vi "Configuracao.Escrita.vi"(8 "error in (no error)":errorcluster) -> (0 "error out":errorcluster)   [LabVIEW 2019]
uses:
  Configuracao.Variaveis.vi
  TelaParametrosTeste/VariaveisParametros.vi
  Relatorio/Relatorio_Variaveis.vi
  <vilib>/Utility/xml.llb/Write to XML File(string).vi
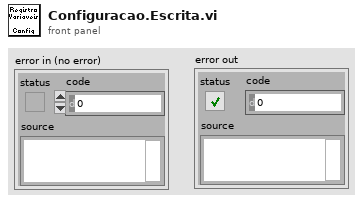
[diagram p1: front panel]
types:
  T1 = enum16{"None", "Continua", "Senoidal", "Quadrada"}
  T2 = cluster{"PicoRotacaoMax":dbl, "PicoRotacaoMin":dbl, "RotacoesMinuto":dbl}
  T3 = cluster{"TempRampas":dbl, "PicoMax":dbl, "TextUnidMed":string}
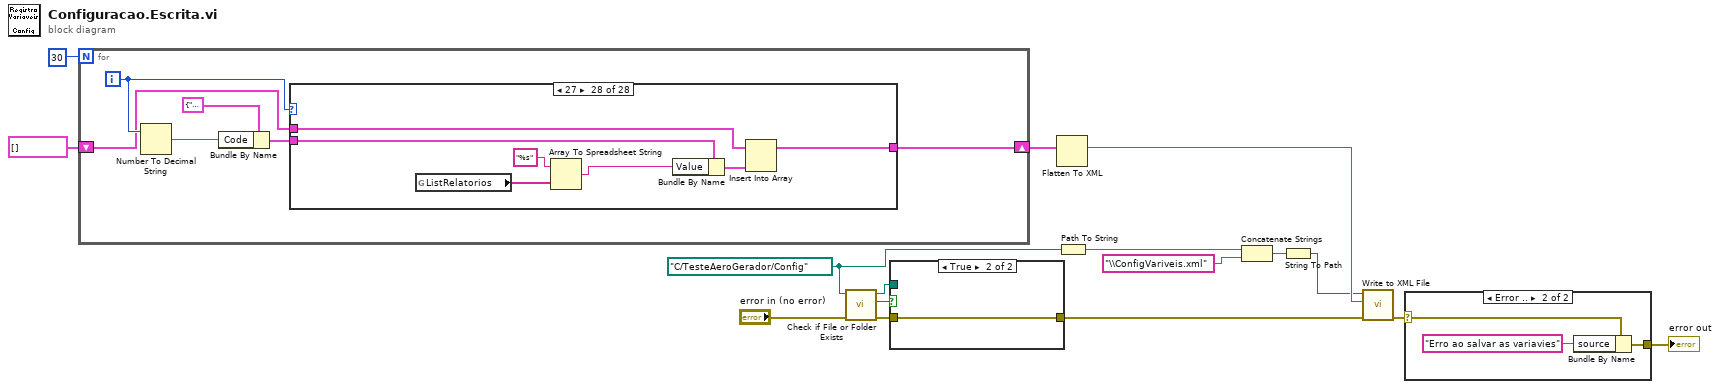
[diagram p0: block diagram]
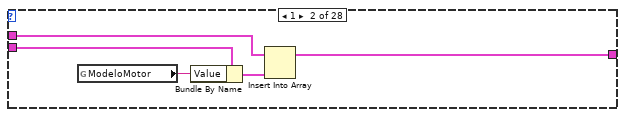
[diagram p4: hidden frame]
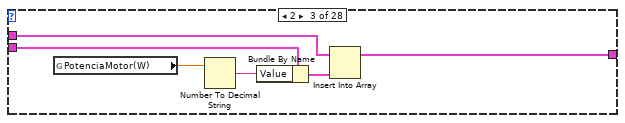
[diagram p5: hidden frame]
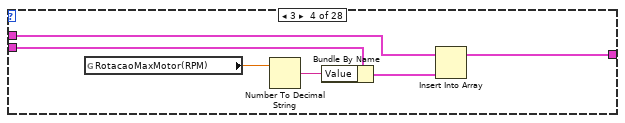
[diagram p6: hidden frame]
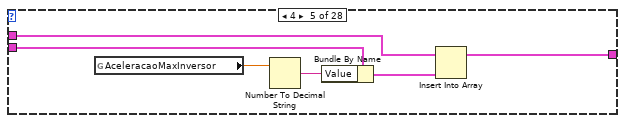
[diagram p7: hidden frame]
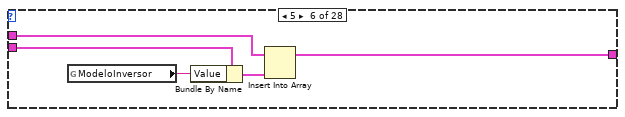
[diagram p8: hidden frame]
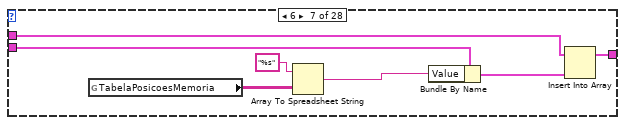
[diagram p9: hidden frame]
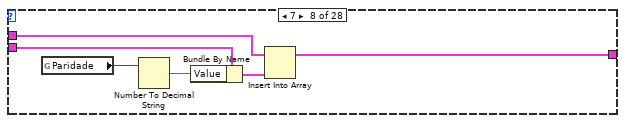
[diagram p10: hidden frame]
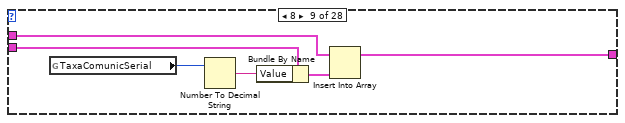
[diagram p11: hidden frame]
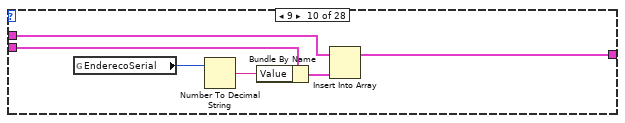
[diagram p12: hidden frame]
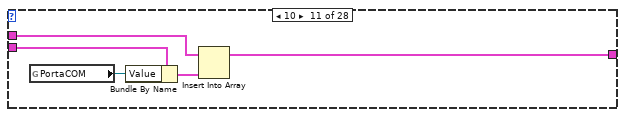
[diagram p13: hidden frame]
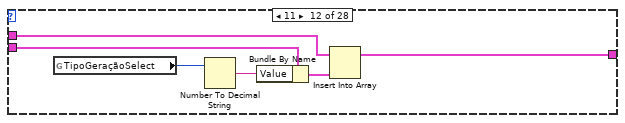
[diagram p14: hidden frame]
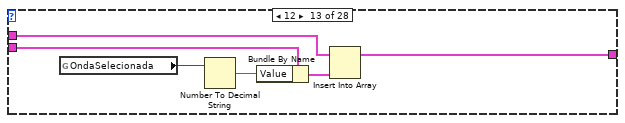
[diagram p15: hidden frame]
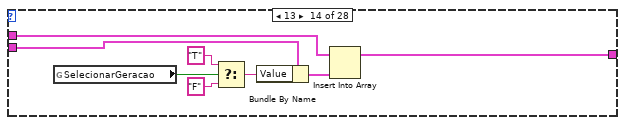
[diagram p16: hidden frame]
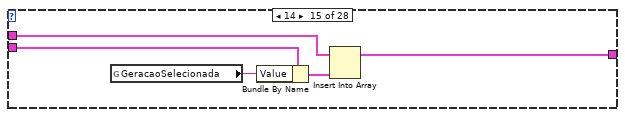
[diagram p17: hidden frame]
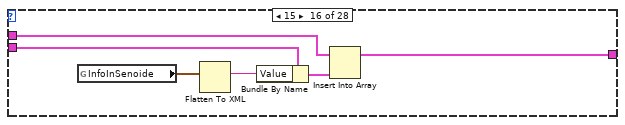
[diagram p18: hidden frame]
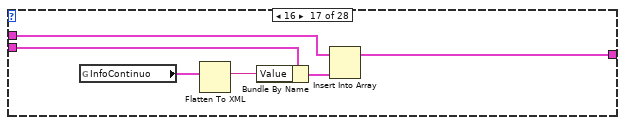
[diagram p19: hidden frame]
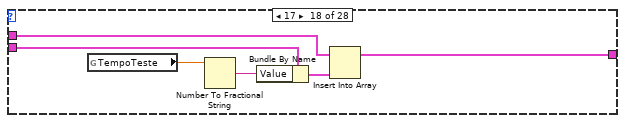
[diagram p20: hidden frame]
diagram:
  w11 = path "C:/TesteAeroGerador/Config" ("XML File Path")
  n1 = for {
    N: 30 -> [_]
    shift-right: [w18] -> w3
    shift-left: cluster{"Code":string, "Value":string}[] [] -> [w19]
    i -> [w20]
    n2 = Number To Decimal String(number=w20) -> (decimal integer string=w21:string)  [unwired: 1 in]
    n3 = Bundle By Name(cluster=cluster{"Code":string, "Value":string} {"Code"="", "Value"=""} ("output cluster"), "Code"=w21) -> (w17:cluster{"Code":string, "Value":string})
    n4 = case shown="27" w20 {
      tunnel: w19 -> [w23 w28 w34 w40 w46 w51 w58 w64 w70 w76 w81 w87 w93 w101 w106 w112 w118 w124 w131 w139 w145 w151 w157 w163 w169 w174 w176 w185]
      tunnel: [w23 w27 w33 w39 w45 w50 w57 w63 w69 w75 w80 w86 w92 w100 w105 w111 w117 w123 w130 w138 w144 w150 w156 w162 w168 w173 w175 w184] -> w18
      tunnel: w17 -> [_ w26 w32 w38 w44 w49 w56 w62 w68 w74 w79 w85 w91 w99 w104 w110 w116 w122 w129 w137 w143 w149 w155 w161 w167 w172 w177 w186]
      frame 0, Default {
      }
      frame 1 {
        n5 = global read "Configuracao.Variaveis.vi" "ModeloMotor"() -> (w25:string)
        n6 = Bundle By Name(cluster=w26, "Value"=w25) -> (w24:cluster{"Code":string, "Value":string})
        n7 = Insert Into Array(array=w28, new element=w24) -> (w27:cluster{"Code":string, "Value":string}[])  [unwired: 1 in]
      }
      frame 2 {
        n8 = global read "Configuracao.Variaveis.vi" "PotenciaMotor(W)"() -> (w30:dbl)
        n9 = Number To Decimal String(number=w30) -> (decimal integer string=w29:string)  [unwired: 1 in]
        n10 = Bundle By Name(cluster=w32, "Value"=w29) -> (w31:cluster{"Code":string, "Value":string})
        n11 = Insert Into Array(array=w34, new element=w31) -> (w33:cluster{"Code":string, "Value":string}[])  [unwired: 1 in]
      }
      frame 3 {
        n12 = global read "Configuracao.Variaveis.vi" "RotacaoMaxMotor(RPM)"() -> (w36:dbl)
        n13 = Number To Decimal String(number=w36) -> (decimal integer string=w35:string)  [unwired: 1 in]
        n14 = Bundle By Name(cluster=w38, "Value"=w35) -> (w37:cluster{"Code":string, "Value":string})
        n15 = Insert Into Array(array=w40, new element=w37) -> (w39:cluster{"Code":string, "Value":string}[])  [unwired: 1 in]
      }
      frame 4 {
        n16 = global read "Configuracao.Variaveis.vi" "AceleracaoMaxInversor"() -> (w42:dbl)
        n17 = Number To Decimal String(number=w42) -> (decimal integer string=w41:string)  [unwired: 1 in]
        n18 = Bundle By Name(cluster=w44, "Value"=w41) -> (w43:cluster{"Code":string, "Value":string})
        n19 = Insert Into Array(array=w46, new element=w43) -> (w45:cluster{"Code":string, "Value":string}[])  [unwired: 1 in]
      }
      frame 5 {
        n20 = global read "Configuracao.Variaveis.vi" "ModeloInversor"() -> (w47:string)
        n21 = Bundle By Name(cluster=w49, "Value"=w47) -> (w48:cluster{"Code":string, "Value":string})
        n22 = Insert Into Array(array=w51, new element=w48) -> (w50:cluster{"Code":string, "Value":string}[])  [unwired: 1 in]
      }
      frame 6 {
        n23 = global read "Configuracao.Variaveis.vi" "TabelaPosicoesMemoria"() -> (w53:string[][])
        n24 = Array To Spreadsheet String(array=w53, 3:"%s" ("format string")) -> (spreadsheet string=w52:string)  [unwired: 1 in]
        n25 = Bundle By Name(cluster=w56, "Value"=w52) -> (w55:cluster{"Code":string, "Value":string})
        n26 = Insert Into Array(array=w58, new element=w55) -> (w57:cluster{"Code":string, "Value":string}[])  [unwired: 1 in]
      }
      frame 7 {
        n27 = global read "Configuracao.Variaveis.vi" "Paridade"() -> (w60:u16)
        n28 = Number To Decimal String(number=w60) -> (decimal integer string=w59:string)  [unwired: 1 in]
        n29 = Bundle By Name(cluster=w62, "Value"=w59) -> (w61:cluster{"Code":string, "Value":string})
        n30 = Insert Into Array(array=w64, new element=w61) -> (w63:cluster{"Code":string, "Value":string}[])  [unwired: 1 in]
      }
      frame 8 {
        n31 = global read "Configuracao.Variaveis.vi" "TaxaComunicSerial"() -> (w66:u32)
        n32 = Number To Decimal String(number=w66) -> (decimal integer string=w65:string)  [unwired: 1 in]
        n33 = Bundle By Name(cluster=w68, "Value"=w65) -> (w67:cluster{"Code":string, "Value":string})
        n34 = Insert Into Array(array=w70, new element=w67) -> (w69:cluster{"Code":string, "Value":string}[])  [unwired: 1 in]
      }
      frame 9 {
        n35 = global read "Configuracao.Variaveis.vi" "EnderecoSerial"() -> (w72:u8)
        n36 = Number To Decimal String(number=w72) -> (decimal integer string=w71:string)  [unwired: 1 in]
        n37 = Bundle By Name(cluster=w74, "Value"=w71) -> (w73:cluster{"Code":string, "Value":string})
        n38 = Insert Into Array(array=w76, new element=w73) -> (w75:cluster{"Code":string, "Value":string}[])  [unwired: 1 in]
      }
      frame 10 {
        n39 = global read "Configuracao.Variaveis.vi" "PortaCOM"() -> (w77:refnum<visa-resource-name>)
        n40 = Bundle By Name(cluster=w79, "Value"=w77) -> (w78:cluster{"Code":string, "Value":string})
        n41 = Insert Into Array(array=w81, new element=w78) -> (w80:cluster{"Code":string, "Value":string}[])  [unwired: 1 in]
      }
      frame 11 {
        n42 = global read "VariaveisParametros.vi" "TipoGeraçãoSelect"() -> (w83:u16)
        n43 = Number To Decimal String(number=w83) -> (decimal integer string=w82:string)  [unwired: 1 in]
        n44 = Bundle By Name(cluster=w85, "Value"=w82) -> (w84:cluster{"Code":string, "Value":string})
        n45 = Insert Into Array(array=w87, new element=w84) -> (w86:cluster{"Code":string, "Value":string}[])  [unwired: 1 in]
      }
      frame 12 {
        n46 = global read "VariaveisParametros.vi" "OndaSelecionada"() -> (w89:T1)
        n47 = Number To Decimal String(number=w89) -> (decimal integer string=w88:string)  [unwired: 1 in]
        n48 = Bundle By Name(cluster=w91, "Value"=w88) -> (w90:cluster{"Code":string, "Value":string})
        n49 = Insert Into Array(array=w93, new element=w90) -> (w92:cluster{"Code":string, "Value":string}[])  [unwired: 1 in]
      }
      frame 13 {
        n50 = global read "VariaveisParametros.vi" "SelecionarGeracao"() -> (w95:bool)
        n51 = Select(t="T", s=w95, f="F") -> (s? t:f=w97:string)
        n52 = Bundle By Name(cluster=w99, "Value"=w97) -> (w98:cluster{"Code":string, "Value":string})
        n53 = Insert Into Array(array=w101, new element=w98) -> (w100:cluster{"Code":string, "Value":string}[])  [unwired: 1 in]
      }
      frame 14 {
        n54 = global read "VariaveisParametros.vi" "GeracaoSelecionada"() -> (w102:string)
        n55 = Bundle By Name(cluster=w104, "Value"=w102) -> (w103:cluster{"Code":string, "Value":string})
        n56 = Insert Into Array(array=w106, new element=w103) -> (w105:cluster{"Code":string, "Value":string}[])  [unwired: 1 in]
      }
      frame 15 {
        n57 = global read "VariaveisParametros.vi" "InfoInSenoide"() -> (w108:T2)
        n58 = Flatten To XML(anything=w108) -> (xml string=w107:string)
        n59 = Bundle By Name(cluster=w110, "Value"=w107) -> (w109:cluster{"Code":string, "Value":string})
        n60 = Insert Into Array(array=w112, new element=w109) -> (w111:cluster{"Code":string, "Value":string}[])  [unwired: 1 in]
      }
      frame 16 {
        n61 = global read "VariaveisParametros.vi" "InfoContinuo"() -> (w114:T3)
        n62 = Flatten To XML(anything=w114) -> (xml string=w113:string)
        n63 = Bundle By Name(cluster=w116, "Value"=w113) -> (w115:cluster{"Code":string, "Value":string})
        n64 = Insert Into Array(array=w118, new element=w115) -> (w117:cluster{"Code":string, "Value":string}[])  [unwired: 1 in]
      }
      frame 17 {
        n65 = global read "VariaveisParametros.vi" "TempoTeste"() -> (w120:dbl)
        n66 = Number To Fractional String(number=w120) -> (F-format string=w119:string)  [unwired: 3 in]
        n67 = Bundle By Name(cluster=w122, "Value"=w119) -> (w121:cluster{"Code":string, "Value":string})
        n68 = Insert Into Array(array=w124, new element=w121) -> (w123:cluster{"Code":string, "Value":string}[])  [unwired: 1 in]
      }
      frame 18 {
        n69 = global read "VariaveisParametros.vi" "ListaMedicaoPorta"() -> (w126:string[][])
        n70 = Array To Spreadsheet String(array=w126, 3:"%s" ("format string")) -> (spreadsheet string=w125:string)  [unwired: 1 in]
        n71 = Bundle By Name(cluster=w129, "Value"=w125) -> (w128:cluster{"Code":string, "Value":string})
        n72 = Insert Into Array(array=w131, new element=w128) -> (w130:cluster{"Code":string, "Value":string}[])  [unwired: 1 in]
      }
      frame 19 {
        n73 = global read "VariaveisParametros.vi" "Pontos"() -> (w133:dbl[])
        n74 = Number To Fractional String(number=w133) -> (F-format string=w132:string[])  [unwired: 3 in]
        n75 = Array To Spreadsheet String(array=w132, 3:"%s" ("format string")) -> (spreadsheet string=w134:string)  [unwired: 1 in]
        n76 = Bundle By Name(cluster=w137, "Value"=w134) -> (w136:cluster{"Code":string, "Value":string})
        n77 = Insert Into Array(array=w139, new element=w136) -> (w138:cluster{"Code":string, "Value":string}[])  [unwired: 1 in]
      }
      frame 20 {
        n78 = global read "VariaveisParametros.vi" "TempoEntrePontos"() -> (w141:dbl)
        n79 = Number To Fractional String(number=w141) -> (F-format string=w140:string)  [unwired: 3 in]
        n80 = Bundle By Name(cluster=w143, "Value"=w140) -> (w142:cluster{"Code":string, "Value":string})
        n81 = Insert Into Array(array=w145, new element=w142) -> (w144:cluster{"Code":string, "Value":string}[])  [unwired: 1 in]
      }
      frame 21 {
        n82 = global read "VariaveisParametros.vi" "TempoAquisicao"() -> (w147:dbl)
        n83 = Number To Fractional String(number=w147) -> (F-format string=w146:string)  [unwired: 3 in]
        n84 = Bundle By Name(cluster=w149, "Value"=w146) -> (w148:cluster{"Code":string, "Value":string})
        n85 = Insert Into Array(array=w151, new element=w148) -> (w150:cluster{"Code":string, "Value":string}[])  [unwired: 1 in]
      }
      frame 22 {
        n86 = global read "VariaveisParametros.vi" "TaxaTransmissãoDados"() -> (w153:dbl)
        n87 = Number To Fractional String(number=w153) -> (F-format string=w152:string)  [unwired: 3 in]
        n88 = Bundle By Name(cluster=w155, "Value"=w152) -> (w154:cluster{"Code":string, "Value":string})
        n89 = Insert Into Array(array=w157, new element=w154) -> (w156:cluster{"Code":string, "Value":string}[])  [unwired: 1 in]
      }
      frame 23 {
        n90 = global read "Configuracao.Variaveis.vi" "RotacaoMaxAeroGerador"() -> (w158:dbl)
        n91 = Number To Fractional String(number=w158) -> (F-format string=w159:string)  [unwired: 3 in]
        n92 = Bundle By Name(cluster=w161, "Value"=w159) -> (w160:cluster{"Code":string, "Value":string})
        n93 = Insert Into Array(array=w163, new element=w160) -> (w162:cluster{"Code":string, "Value":string}[])  [unwired: 1 in]
      }
      frame 24 {
        n94 = global read "Configuracao.Variaveis.vi" "RotacaoMaxSistema"() -> (w164:dbl)
        n95 = Number To Fractional String(number=w164) -> (F-format string=w165:string)  [unwired: 3 in]
        n96 = Bundle By Name(cluster=w167, "Value"=w165) -> (w166:cluster{"Code":string, "Value":string})
        n97 = Insert Into Array(array=w169, new element=w166) -> (w168:cluster{"Code":string, "Value":string}[])  [unwired: 1 in]
      }
      frame 25 {
        n98 = global read "Configuracao.Variaveis.vi" "ModeloAeroGerador"() -> (w170:string)
        n99 = Bundle By Name(cluster=w172, "Value"=w170) -> (w171:cluster{"Code":string, "Value":string})
        n100 = Insert Into Array(array=w174, new element=w171) -> (w173:cluster{"Code":string, "Value":string}[])  [unwired: 1 in]
      }
      frame 26 {
        n101 = global read "Configuracao.Variaveis.vi" "PotenciaAero"() -> (w178:dbl)
        n102 = Number To Fractional String(number=w178) -> (F-format string=w179:string)  [unwired: 3 in]
        n103 = Bundle By Name(cluster=w177, "Value"=w179) -> (w180:cluster{"Code":string, "Value":string})
        n104 = Insert Into Array(array=w176, new element=w180) -> (w175:cluster{"Code":string, "Value":string}[])  [unwired: 1 in]
      }
      frame 27 {
        n105 = global read "Relatorio_Variaveis.vi" "ListRelatorios"() -> (w181:string[])
        n106 = Array To Spreadsheet String(array=w181, 3:"%s" ("format string")) -> (spreadsheet string=w182:string)  [unwired: 1 in]
        n107 = Bundle By Name(cluster=w186, "Value"=w182) -> (w187:cluster{"Code":string, "Value":string})
        n108 = Insert Into Array(array=w185, new element=w187) -> (w184:cluster{"Code":string, "Value":string}[])  [unwired: 1 in]
      }
    }
  }
  n109 = call <vilib>:"Check if File or Folder Exists.vi"("error in (no error)"="error in (no error)", "path"=w11) -> ("error out"=w15:errorcluster, "file or folder exists?"=w16:bool, "dup path"=w6:path)  [unwired: 7 in]
  n110 = case shown="True" w16 {
    tunnel: w6 -> [w190 _]
    tunnel: w15 -> [w189 w191]
    tunnel: [w188 w191] -> w13
    frame False {
      n111 = Create Folder(path (use dialog)=w190, error in=w189) -> (error out=w188:errorcluster)  [unwired: 1 in, 2 out]
    }
    frame True {
    }
  }
  n112 = Flatten To XML(anything=w3) -> (xml string=w12:string)
  n113 = Path To String(path=w11) -> (string=w10:string)
  n114 = Concatenate Strings(w10, "\\ConfigVariveis.xml") -> (w8:string)
  n115 = String To Path(string=w8) -> (path=w7:path)
  n116 = call-poly <vilib>:"Write to XML File.vi"("error in (no error)"=w13, "XML Input"=w12, "XML File Path"=w7) -> ("error out"=w2:errorcluster)  [unwired: 6 in, 2 out]
  n117 = case shown="Error .." w2 {
    selector: w2 -> [w192 w195]
    tunnel: [w192 w193] -> w1
    frame No Error {
    }
    frame Error {
      n118 = Bundle By Name(cluster=w195, "source"="Erro ao salvar as variavies") -> (w193:errorcluster)
    }
  }
  "error out" <- w1
